vi "MACBIN Copy Fork From File__ogtk.vi"(4 "length":i32, 5 "error out":errorcluster, 7 "fork Refnum":refnum<file>, 8 "macbinary Refnum":refnum<file>) -> (0 "error out":errorcluster, 2 "forkname out":path, 3 "macbinary Refnum out":refnum<file>)   [LabVIEW 2018]
panel:
  # "Please visit http://www.OpenG.org to learn about the\nOpen Source LabVIEW software movement.\n\nNOTICE -- YOU MUST LEAVE THIS NOTICE IN PLACE.  PER THE TERMS OF THE LICENSE BELOW, YOU MAY SUBLICENSE THIS SOFTWARE \nIN ANY WAY THAT DOES NOT CONFLICT WITH THIS LICENSE.\n\n### BSD License (http://www.opensource.org/licenses/bsd-license.php) Begin ###\n \nCopyright (C) 2002 Christophe Salzmann christophe.salzmann@epfl.ch\nCopyright (C) 2002 Rolf Kalbermatter rolf.kalbermatter@citengineering.com\n\nAll rights reserved.\n\nRedistribution and use in source and binary forms, with or without modification, are permitted provided that the following conditions are met:\n\n    * Redistributions of source code must retain the above copyright notice, this list of conditions and the following disclaimer.\n    * Redistributions in binary form must reproduce the above copyright notice, this list of conditions and the following disclaimer in the \n       documentation and/or other materials provided with the distribution.\n    * Neither the name of SciWare, James Kring, Inc., nor the names of its contributors may be used to endorse or promote products derived \n       from this software without specific prior written permission.\n\nTHIS SOFTWARE IS PROVIDED BY THE COPYRIGHT HOLDERS AND CONTRIBUTORS \"AS IS\" AND ANY EXPRESS OR IMPLIED WARRANTIES, \nINCLUDING, BUT NOT LIMITED TO, THE IMPLIED WARRANTIES OF MERCHANTABILITY AND FITNESS FOR A PARTICULAR PURPOSE ARE \nDISCLAIMED. IN NO EVENT SHALL THE COPYRIGHT OWNER OR CONTRIBUTORS BE LIABLE FOR ANY DIRECT, INDIRECT, INCIDENTAL,\n SPECIAL, EXEMPLARY, OR CONSEQUENTIAL DAMAGES (INCLUDING, BUT NOT LIMITED TO, PROCUREMENT OF SUBSTITUTE GOODS OR \nSERVICES; LOSS OF USE, DATA, OR PROFITS; OR BUSINESS INTERRUPTION) HOWEVER CAUSED AND ON ANY THEORY OF LIABILITY, \nWHETHER IN CONTRACT, STRICT LIABILITY, OR TORT (INCLUDING NEGLIGENCE OR OTHERWISE) ARISING IN ANY WAY OUT OF THE USE \nOF THIS SOFTWARE, EVEN IF ADVISED OF THE POSSIBILITY OF SUCH DAMAGE.\n\n### BSD License End ###"
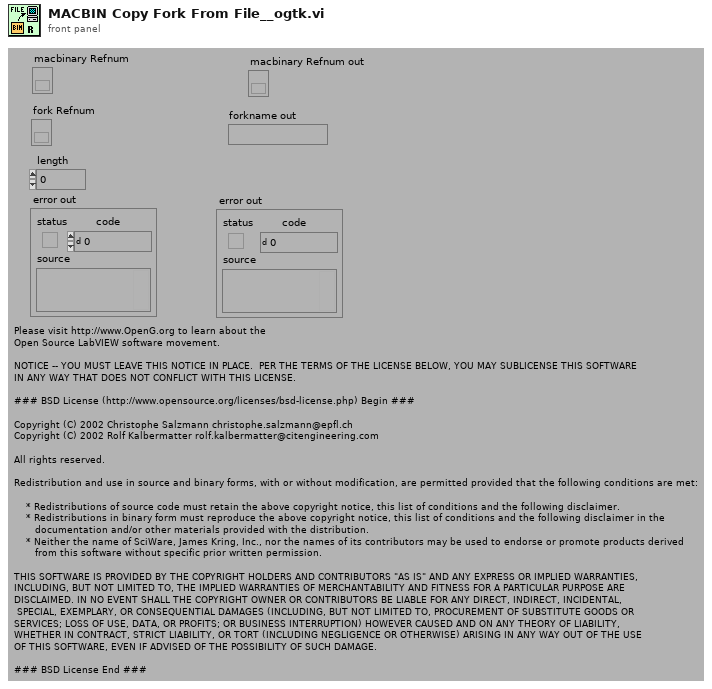
[diagram p1: front panel]
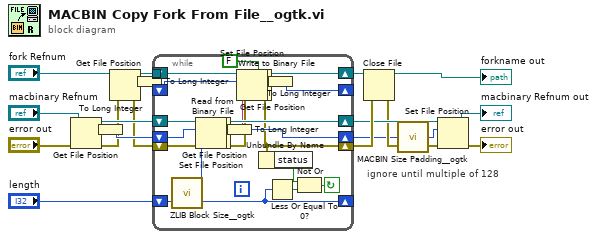
[diagram p0: block diagram]
diagram:
  # "ignore until multiple of 128"
  n1 = Get File Position(4:"error out", 7:"macbinary Refnum") -> (0:w4:errorcluster, 2:w1:i64, 3:w17:refnum<file>)
  n2 = To Long Integer(number=w1) -> (32bit integer=w18:i32)
  n3 = Get File Position(4:w4, 7:"fork Refnum") -> (0:w5:errorcluster, 2:w2:i64, 3:w6:refnum<file>)
  n4 = To Long Integer(number=w2) -> (32bit integer=w8:i32)
  n5 = while {
    tunnel: [w36] -> _
    shift-left: "length" -> [w44]
    shift-right: [w40] -> _
    shift-left: w6 -> [w36]
    shift-right: [w35] -> w20
    shift-left: w8 -> [w34]
    shift-right: [w45] -> _
    shift-left: w17 -> [w48]
    shift-right: [w47] -> w14
    shift-left: w5 -> [w46]
    shift-right: [w37] -> w21
    shift-left: w18 -> [w50]
    shift-right: [w49] -> w10
    stop <- w43 continue-if-true
    n6 = call <userlib>:"ZLIB Block Size__ogtk.vi"("length in"=w44) -> ("length rem"=w40:u32, "block len"=w39:u32)  [unwired: 1 in]
    n7 = Set File Position(offset (in bytes) (0)=w50, refnum=w48, error in=w46) -> (refnum out=w26:refnum<file>, error out=w25:errorcluster)  [unwired: 1 in]
    n8 = Read from Binary File(8:w25, 10:w39, 11:w26) -> (0:w23:errorcluster, 2:w33:string, 3:w24:refnum<file>)  [unwired: 3 in, 1 out]
    n9 = Get File Position(4:w23, 7:w24) -> (0:w38:errorcluster, 2:w22:i64, 3:w47:refnum<file>)
    n10 = To Long Integer(number=w22) -> (32bit integer=w49:i32)
    n11 = Set File Position(offset (in bytes) (0)=w34, refnum=w36, error in=w38) -> (refnum out=w32:refnum<file>, error out=w31:errorcluster)  [unwired: 1 in]
    n12 = Write to Binary File(file (use dialog)=w32, data=w33, error in=w31, 5:FALSE ("prepend array or string size? (T)")) -> (refnum out=w30:refnum<file>, error out=w29:errorcluster)  [unwired: 2 in, 1 out]
    n13 = Get File Position(4:w29, 7:w30) -> (0:w37:errorcluster, 2:w28:i64, 3:w35:refnum<file>)
    n14 = Unbundle By Name(w37) -> ("status"=w42:bool)
    n15 = To Long Integer(number=w28) -> (32bit integer=w45:i32)
    n16 = Less Or Equal To 0?(x=w40) -> (x <= 0?=w41:bool)
    n17 = Not Or(1:w41, 2:w42) -> (0:w43:bool)
  }
  n18 = Close File(refnum=w20, error in=w21) -> (path=→"forkname out":path, error out=w13:errorcluster)
  n19 = call <userlib>:"MACBIN Size Padding__ogtk.vi"("length"=w10) -> ("padded length"=w9:i32)  [unwired: 4 in]
  n20 = Set File Position(offset (in bytes) (0)=w9, refnum=w14, error in=w13) -> (refnum out=→"macbinary Refnum out":refnum<file>, error out=→"error out":errorcluster)  [unwired: 1 in]
